vi "Log.vi"(8 "error in (no error)":errorcluster, 10 "Log Text":string, 11 "Directory":path) -> (0 "error out":errorcluster)   [LabVIEW 2020, in "Library Builder.lvlib"]
uses:
  Library Builder.lvlib
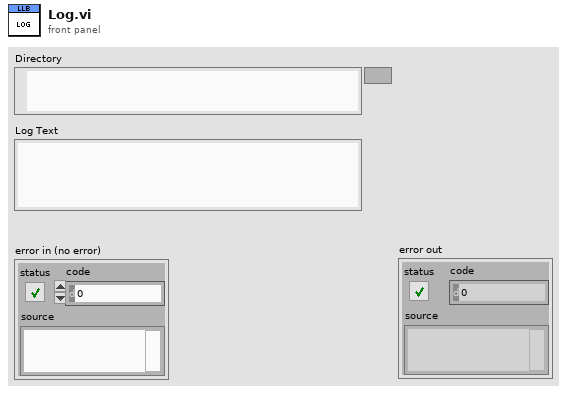
[diagram p1: front panel]
types:
  T1 = enum16{"open", "replace", "create", "open or create", "replace or create", "replace or create with confirmation"}
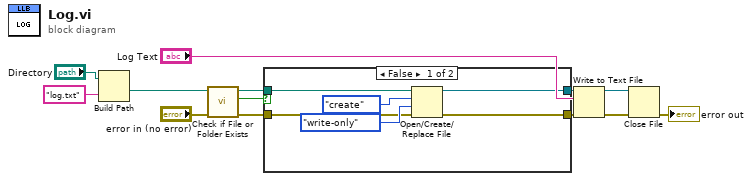
[diagram p0: block diagram]
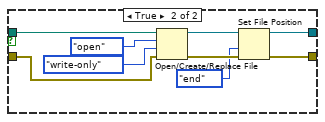
[diagram p2: hidden frame]
diagram:
  n1 = Build Path(base path="Directory", name or relative path="log.txt" ("time format string (%c)")) -> (appended path=w1:path)
  n2 = call <vilib>:"Check if File or Folder Exists.vi"("error in (no error)"="error in (no error)", "path"=w1) -> ("error out"=w5:errorcluster, "file or folder exists?"=w4:bool, "dup path"=w6:path)  [unwired: 7 in]
  n3 = case shown="False" w4 {
    tunnel: [w17 w21] -> w12
    tunnel: [w16 w22] -> w11
    tunnel: w6 -> [w15 w26]
    tunnel: w5 -> [w14 w25]
    frame False {
      n4 = Open/Create/Replace File(file path (use dialog)=w15, error in=w14, operation (0:open)=T1."create", access (0:read/write)=enum16{"read/write", "read-only", "write-only"}."write-only") -> (refnum out=w16:refnum<file>, error out=w17:errorcluster)  [unwired: 2 in, 1 out]
    }
    frame True {
      n5 = Open/Create/Replace File(file path (use dialog)=w26, error in=w25, operation (0:open)=T1."open", access (0:read/write)=enum16{"read/write", "read-only", "write-only"}."write-only") -> (refnum out=w24:refnum<file>, error out=w23:errorcluster)  [unwired: 2 in, 1 out]
      n6 = Set File Position(refnum=w24, from (0:start)=enum16{"start", "end", "current"}."end", error in=w23) -> (refnum out=w22:refnum<file>, error out=w21:errorcluster)  [unwired: 1 in]
    }
  }
  n7 = Write to Text File(file (use dialog)=w11, text="Log Text", error in=w12) -> (refnum out=w10:refnum<file>, error out=w9:errorcluster)  [unwired: 1 in, 1 out]
  n8 = Close File(refnum=w10, error in=w9) -> (error out=→"error out":errorcluster)  [unwired: 1 out]
